vi "Find All.vi"(8 "Error In":errorcluster, 11 "VI In":refnum<vi>) -> (0 "Error Out":errorcluster, 2 "Grave Sites":refnum<vi>[](array[refnum]), 3 "VI Out":refnum<vi>)   [LabVIEW 2017, in "Eulogy.lvlib"]
doc: "Finds all grave sites in the VI."
uses:
  Eulogy.lvlib
  <vilib>/Utility/traverseref.llb/TRef TravTarget.ctl
  <vilib>/Utility/traverseref.llb/VI Scripting - Traverse.lvlib
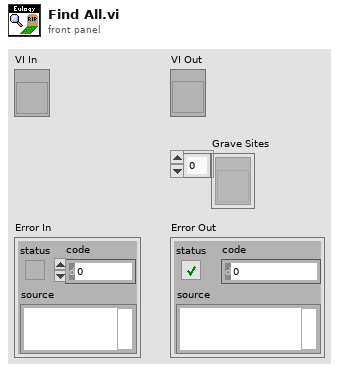
[diagram p1: front panel]
types:
  T1 = typedef "TRef TravTarget.ctl" = enum16{"FP", "BD", "Other"}
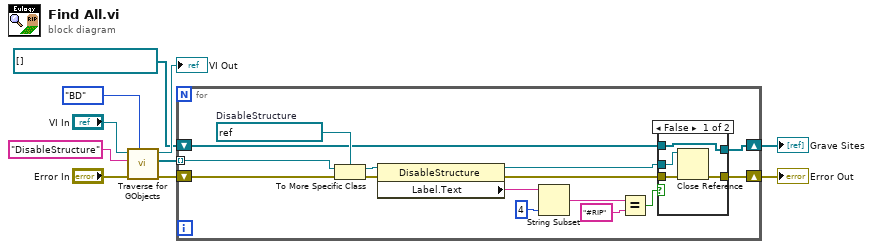
[diagram p0: block diagram]
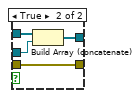
[diagram p2: hidden frame]
diagram:
  n1 = call <vilib>:"Traverse for GObjects.vi"("Traverse Target"=TRef_TravTarget."BD", "error in (no error)"="Error In", "Class Name"="DisableStructure", "VI Refnum"="VI In") -> ("error out"=w6:errorcluster, "References"=w5:refnum<vi>[], "dup VI Refnum"=→"VI Out":refnum<vi>)  [unwired: 4 in, 1 out]
  n2 = for {
    shift-right: [w15] -> w3
    shift-left: w6 -> [w25]
    tunnel: w5 -> [w24] mode=indexing
    shift-right: [w11] -> w1
    shift-left: refnum<vi>[] [] -> [w12]
    w21 = refnum<vi> refnum  # DisableStructure
    n3 = To More Specific Class(target class=w21, reference=w24, error in=w25) -> (specific class reference=w22:refnum<vi>, error out=w23:errorcluster)
    n4 = property class="DisableStructure"(reference=w22, error in=w23) -> (reference out=w13:refnum<vi>, error out=w16:errorcluster, "Label.Text"=w20:string)
    n5 = String Subset(string=w20, length (rest)=4 ("length (rest)")) -> (substring=w18:string)  [unwired: 1 in]
    n6 = Equal?(x=w18, y="#RIP") -> (x = y?=w14:bool)
    n7 = case shown="False" w14 {
      tunnel: w16 -> [w29 w33]
      tunnel: [w28 w33] -> w15
      tunnel: w13 -> [w27 w31]
      tunnel: w12 -> [w26 w32]
      tunnel: [w26 w30] -> w11
      frame False {
        n8 = Close Reference(reference=w27, error in (no error)=w29) -> (error out=w28:errorcluster)
      }
      frame True {
        n9 = Build Array (concatenate)(w32, w31) -> (w30:refnum<vi>[])
      }
    }
  }
  "Error Out" <- w3
  "Grave Sites" <- w1
